vi "bumper b.vi"() -> ()   [LabVIEW 2013]
uses:
  <vilib>/NXT/Subs/MotorOutput.ctl
  <vilib>/NXT/Block Support/NXT_InputPort.ctl
panel:
  out "Output Ports (A & B) 34":T1=4 items=["Port A"=0, "Port B"=1, "Port C"=2, "Ports A & B"=4, "Ports A & C"=5, "Ports B & C"=6, "All Ports"=3]
  out "Output Port (All Ports) 15":T1=3 items=["Port A"=0, "Port B"=1, "Port C"=2, "Ports A & B"=4, "Ports A & C"=5, "Ports B & C"=6, "All Ports"=3]
  out "Output Ports (A & B) 33":T1=4 items=["Port A"=0, "Port B"=1, "Port C"=2, "Ports A & B"=4, "Ports A & C"=5, "Ports B & C"=6, "All Ports"=3]
  out "Output Ports (A & B) 32":T1=4 items=["Port A"=0, "Port B"=1, "Port C"=2, "Ports A & B"=4, "Ports A & C"=5, "Ports B & C"=6, "All Ports"=3]
  out "Output Port (All Ports) 14":T1=3 items=["Port A"=0, "Port B"=1, "Port C"=2, "Ports A & B"=4, "Ports A & C"=5, "Ports B & C"=6, "All Ports"=3]
  out "Output Ports (A & B) 31":T1=4 items=["Port A"=0, "Port B"=1, "Port C"=2, "Ports A & B"=4, "Ports A & C"=5, "Ports B & C"=6, "All Ports"=3]
  out "Output Ports (A & B) 30":T1=4 items=["Port A"=0, "Port B"=1, "Port C"=2, "Ports A & B"=4, "Ports A & C"=5, "Ports B & C"=6, "All Ports"=3]
  out "Output Port (All Ports) 13":T1=3 items=["Port A"=0, "Port B"=1, "Port C"=2, "Ports A & B"=4, "Ports A & C"=5, "Ports B & C"=6, "All Ports"=3]
  out "Output Ports (A & B) 29":T1=4 items=["Port A"=0, "Port B"=1, "Port C"=2, "Ports A & B"=4, "Ports A & C"=5, "Ports B & C"=6, "All Ports"=3]
  out "Output Ports (A & B) 28":T1=4 items=["Port A"=0, "Port B"=1, "Port C"=2, "Ports A & B"=4, "Ports A & C"=5, "Ports B & C"=6, "All Ports"=3]
  out "Output Port (All Ports) 12":T1=3 items=["Port A"=0, "Port B"=1, "Port C"=2, "Ports A & B"=4, "Ports A & C"=5, "Ports B & C"=6, "All Ports"=3]
  out "Output Ports (A & B) 27":T1=4 items=["Port A"=0, "Port B"=1, "Port C"=2, "Ports A & B"=4, "Ports A & C"=5, "Ports B & C"=6, "All Ports"=3]
  out "Output Ports (A & B) 26":T1=4 items=["Port A"=0, "Port B"=1, "Port C"=2, "Ports A & B"=4, "Ports A & C"=5, "Ports B & C"=6, "All Ports"=3]
  out "Output Port (All Ports) 11":T1=3 items=["Port A"=0, "Port B"=1, "Port C"=2, "Ports A & B"=4, "Ports A & C"=5, "Ports B & C"=6, "All Ports"=3]
  out "Output Ports (A & B) 25":T1=4 items=["Port A"=0, "Port B"=1, "Port C"=2, "Ports A & B"=4, "Ports A & C"=5, "Ports B & C"=6, "All Ports"=3]
  out "Output Ports (A & B) 24":T1=4 items=["Port A"=0, "Port B"=1, "Port C"=2, "Ports A & B"=4, "Ports A & C"=5, "Ports B & C"=6, "All Ports"=3]
  out "Output Port (All Ports) 10":T1=3 items=["Port A"=0, "Port B"=1, "Port C"=2, "Ports A & B"=4, "Ports A & C"=5, "Ports B & C"=6, "All Ports"=3]
  out "Output Ports (A & B) 23":T1=4 items=["Port A"=0, "Port B"=1, "Port C"=2, "Ports A & B"=4, "Ports A & C"=5, "Ports B & C"=6, "All Ports"=3]
  out "Output Ports (A & B) 22":T1=4 items=["Port A"=0, "Port B"=1, "Port C"=2, "Ports A & B"=4, "Ports A & C"=5, "Ports B & C"=6, "All Ports"=3]
  out "Output Port (All Ports) 9":T1=3 items=["Port A"=0, "Port B"=1, "Port C"=2, "Ports A & B"=4, "Ports A & C"=5, "Ports B & C"=6, "All Ports"=3]
  out "Output Ports (A & B) 21":T1=4 items=["Port A"=0, "Port B"=1, "Port C"=2, "Ports A & B"=4, "Ports A & C"=5, "Ports B & C"=6, "All Ports"=3]
  out "Output Ports (A & B) 20":T1=4 items=["Port A"=0, "Port B"=1, "Port C"=2, "Ports A & B"=4, "Ports A & C"=5, "Ports B & C"=6, "All Ports"=3]
  out "Output Port (All Ports) 8":T1=3 items=["Port A"=0, "Port B"=1, "Port C"=2, "Ports A & B"=4, "Ports A & C"=5, "Ports B & C"=6, "All Ports"=3]
  out "Output Ports (A & B) 19":T1=4 items=["Port A"=0, "Port B"=1, "Port C"=2, "Ports A & B"=4, "Ports A & C"=5, "Ports B & C"=6, "All Ports"=3]
  out "Output Ports (A & B) 18":T1=4 items=["Port A"=0, "Port B"=1, "Port C"=2, "Ports A & B"=4, "Ports A & C"=5, "Ports B & C"=6, "All Ports"=3]
  out "Output Port (All Ports) 7":T1=3 items=["Port A"=0, "Port B"=1, "Port C"=2, "Ports A & B"=4, "Ports A & C"=5, "Ports B & C"=6, "All Ports"=3]
  out "Output Ports (A & B) 17":T1=4 items=["Port A"=0, "Port B"=1, "Port C"=2, "Ports A & B"=4, "Ports A & C"=5, "Ports B & C"=6, "All Ports"=3]
  out "Output Ports (A & B) 16":T1=4 items=["Port A"=0, "Port B"=1, "Port C"=2, "Ports A & B"=4, "Ports A & C"=5, "Ports B & C"=6, "All Ports"=3]
  out "Output Port (All Ports) 6":T1=3 items=["Port A"=0, "Port B"=1, "Port C"=2, "Ports A & B"=4, "Ports A & C"=5, "Ports B & C"=6, "All Ports"=3]
  out "Output Ports (A & B) 15":T1=4 items=["Port A"=0, "Port B"=1, "Port C"=2, "Ports A & B"=4, "Ports A & C"=5, "Ports B & C"=6, "All Ports"=3]
  out "Output Ports (A & B) 14":T1=4 items=["Port A"=0, "Port B"=1, "Port C"=2, "Ports A & B"=4, "Ports A & C"=5, "Ports B & C"=6, "All Ports"=3]
  out "Output Port (All Ports) 5":T1=3 items=["Port A"=0, "Port B"=1, "Port C"=2, "Ports A & B"=4, "Ports A & C"=5, "Ports B & C"=6, "All Ports"=3]
  out "Output Ports (A & B) 13":T1=4 items=["Port A"=0, "Port B"=1, "Port C"=2, "Ports A & B"=4, "Ports A & C"=5, "Ports B & C"=6, "All Ports"=3]
  out "Output Ports (A & B) 9":T1=4 items=["Port A"=0, "Port B"=1, "Port C"=2, "Ports A & B"=4, "Ports A & C"=5, "Ports B & C"=6, "All Ports"=3]
  out "Output Port (All Ports) 4":T1=3 items=["Port A"=0, "Port B"=1, "Port C"=2, "Ports A & B"=4, "Ports A & C"=5, "Ports B & C"=6, "All Ports"=3]
  out "Output Ports (A & B) 11":T1=4 items=["Port A"=0, "Port B"=1, "Port C"=2, "Ports A & B"=4, "Ports A & C"=5, "Ports B & C"=6, "All Ports"=3]
  out "Output Port (All Ports) 3":T1=3 items=["Port A"=0, "Port B"=1, "Port C"=2, "Ports A & B"=4, "Ports A & C"=5, "Ports B & C"=6, "All Ports"=3]
  out "Output Ports (A & B) 12":T1=4 items=["Port A"=0, "Port B"=1, "Port C"=2, "Ports A & B"=4, "Ports A & C"=5, "Ports B & C"=6, "All Ports"=3]
  out "Output Ports (A & B) 10":T1=4 items=["Port A"=0, "Port B"=1, "Port C"=2, "Ports A & B"=4, "Ports A & C"=5, "Ports B & C"=6, "All Ports"=3]
  out "Output Ports (A & B) 5":T1=4 items=["Port A"=0, "Port B"=1, "Port C"=2, "Ports A & B"=4, "Ports A & C"=5, "Ports B & C"=6, "All Ports"=3]
  out "touch right":bool
  out "touch left":bool
  in  "threshold steer":dbl=0.2
  out "norm dist":dbl
  out "right dist":i16
  out "left dist":i16
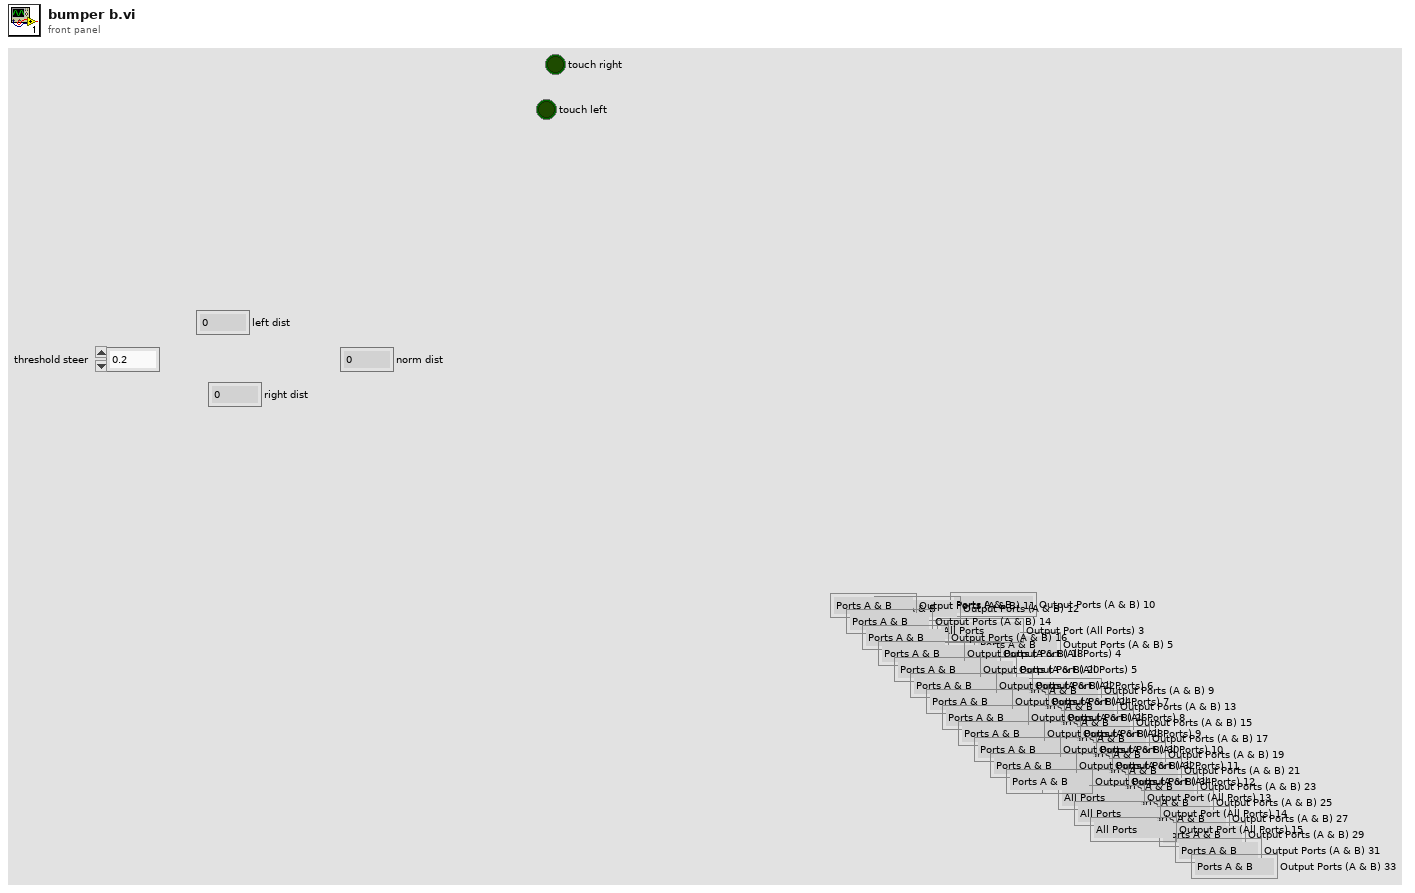
[diagram p1: front panel]
types:
  T1 = typedef "MotorOutput.ctl" = u8
  T2 = typedef "NXT_InputPort.ctl" = u32
  T3 = typedef "LVHSConnector.ctl" = refnum<class "BrickReference.lvclass">
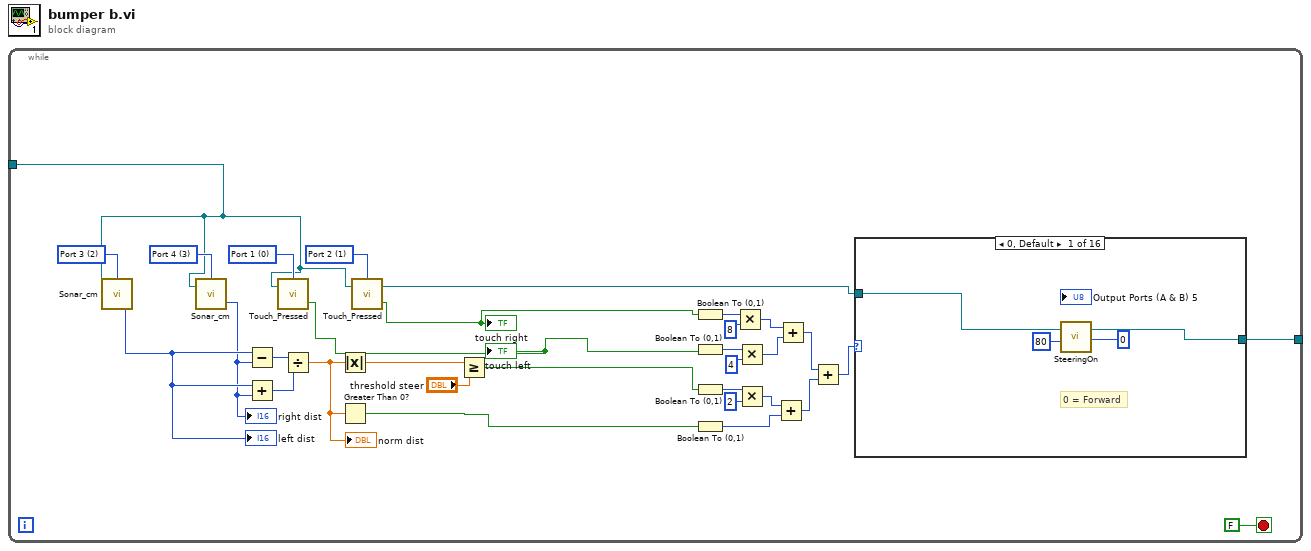
[diagram p0: block diagram]
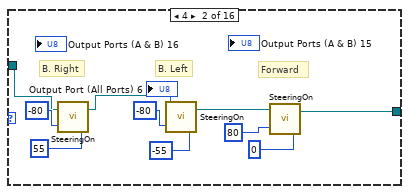
[diagram p2: hidden frame]
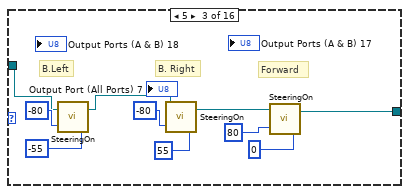
[diagram p3: hidden frame]
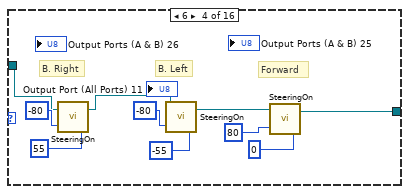
[diagram p4: hidden frame]
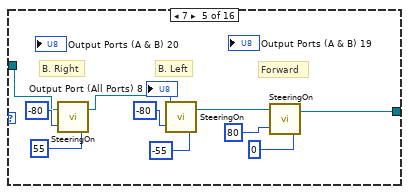
[diagram p5: hidden frame]
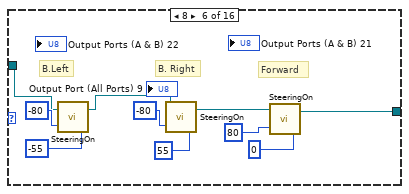
[diagram p6: hidden frame]
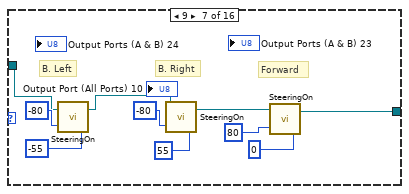
[diagram p7: hidden frame]
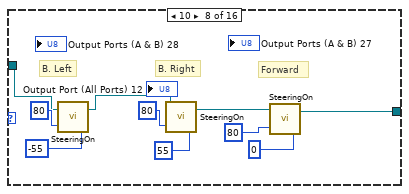
[diagram p8: hidden frame]
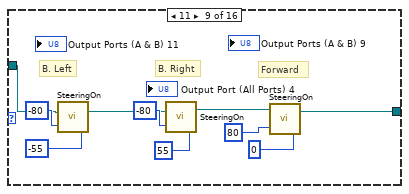
[diagram p9: hidden frame]
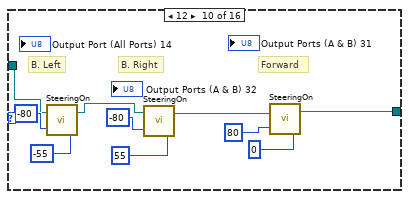
[diagram p10: hidden frame]
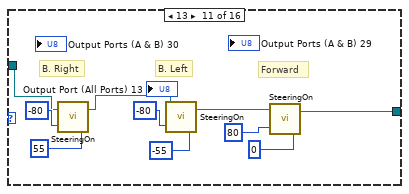
[diagram p11: hidden frame]
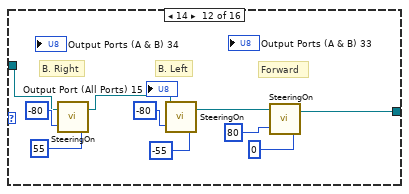
[diagram p12: hidden frame]
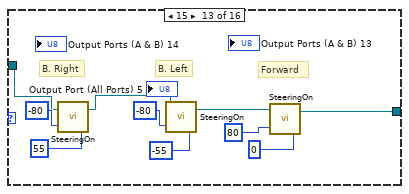
[diagram p13: hidden frame]
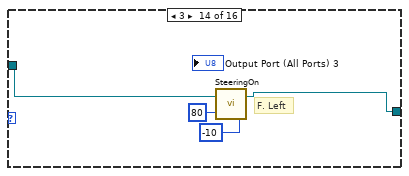
[diagram p14: hidden frame]
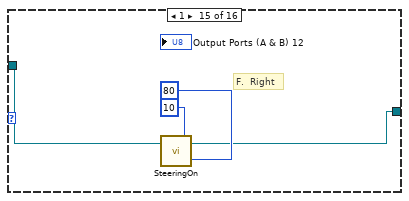
[diagram p15: hidden frame]
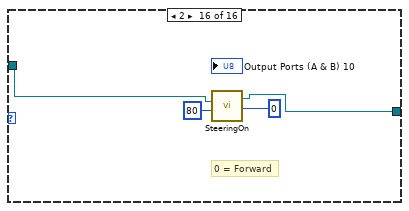
[diagram p16: hidden frame]
diagram:
  n1 = while {
    tunnel: [w7] -> _
    tunnel: [w1] -> _
    stop <- FALSE stop-if-true
    w22 = T2 1 items=["Port 1", "Port 2", "Port 3", "Port 4"] ("Port (Port 1)")
    w23 = T2 0 items=["Port 1", "Port 2", "Port 3", "Port 4"] ("Port (Port 1)")
    w31 = T2 3 items=["Port 1", "Port 2", "Port 3", "Port 4"] ("Port (Port 4)")
    w32 = T2 2 items=["Port 1", "Port 2", "Port 3", "Port 4"] ("Port (Port 4)")
    n2 = call <vilib>:"Sonar_cm.vi"("Port (Port 4)"=w32) -> ("Distance (cm)"=w30:i16, "NXT/EV3"=w1:T3)  [unwired: 2 in]
    "left dist" <- w30
    n3 = call <vilib>:"Sonar_cm.vi"("NXT/EV3"=w1, "Port (Port 4)"=w31) -> ("Distance (cm)"=w29:i16)  [unwired: 1 in, 1 out]
    "right dist" <- w29
    n4 = Subtract(x=w30, y=w29) -> (x-y=w28:i16)
    n5 = Add(x=w30, y=w29) -> (x+y=w27:i16)
    n6 = call <vilib>:"Touch_Pressed.vi"("NXT/EV3"=w1, "Port (Port 1)"=w23) -> ("Yes / No"=w4:bool)  [unwired: 1 in, 1 out]
    "touch left" <- w4
    n7 = Divide(x=w28, y=w27) -> (x/y=w24:dbl)
    "norm dist" <- w24
    n8 = Absolute Value(x=w24) -> (abs(x)=w26:dbl)
    n9 = Greater Than 0?(x=w24) -> (x > 0?=w9:bool)
    n10 = call <vilib>:"Touch_Pressed.vi"("NXT/EV3"=w1, "Port (Port 1)"=w22) -> ("Yes / No"=w3:bool, "NXT/EV3"=w2:T3)  [unwired: 1 in]
    "touch right" <- w3
    n11 = Greater Or Equal?(x=w26, y="threshold steer") -> (x >= y?=w8:bool)
    n12 = Boolean To (0,1)(Boolean=w3) -> (0, 1=w17:i16)
    n13 = Boolean To (0,1)(Boolean=w4) -> (0, 1=w16:i16)
    n14 = Boolean To (0,1)(Boolean=w8) -> (0, 1=w21:i16)
    n15 = Boolean To (0,1)(Boolean=w9) -> (0, 1=w11:i16)
    n16 = Multiply(x=w17, y=i16 8) -> (x*y=w14:i16)
    n17 = Multiply(x=w16, y=i16 4) -> (x*y=w13:i16)
    n18 = Multiply(x=w21, y=i16 2) -> (x*y=w12:i16)
    n19 = Add(x=w12, y=w11) -> (x+y=w10:i16)
    n20 = Add(x=w14, y=w13) -> (x+y=w15:i16)
    n21 = Add(x=w15, y=w10) -> (x+y=w5:i16)
    n22 = case shown="0, Default" w5 {
      tunnel: w2 -> [w34 w40 w50 w60 w70 w80 w90 w100 w110 w120 w130 w140 w150 w158 w162 w166]
      tunnel: [w33 w37 w47 w57 w67 w77 w87 w97 w107 w117 w127 w137 w147 w157 w161 w165] -> w7
      frame 0, Default {
        # "0 = Forward"
        n23 = call <vilib>:"SteeringOn.vi"("Power (75)"=80, "Steering (100)"=0, "NXT/EV3"=w34) -> ("NXT/EV3"=w33:T3)  [unwired: 1 in]
      }
      frame 4 {
        # "Forward"
        # "B. Left"
        # "B. Right"
        n24 = call <vilib>:"SteeringOn.vi"("Power (75)"=-80, "Steering (100)"=55, "NXT/EV3"=w40) -> ("NXT/EV3"=w39:T3)  [unwired: 1 in]
        n25 = call <vilib>:"SteeringOn.vi"("Power (75)"=-80, "Steering (100)"=-55, "NXT/EV3"=w39) -> ("NXT/EV3"=w38:T3)  [unwired: 1 in]
        n26 = call <vilib>:"SteeringOn.vi"("Power (75)"=80, "Steering (100)"=0, "NXT/EV3"=w38) -> ("NXT/EV3"=w37:T3)  [unwired: 1 in]
      }
      frame 5 {
        # "Forward"
        # "B. Right"
        # "B.Left"
        n27 = call <vilib>:"SteeringOn.vi"("Power (75)"=-80, "Steering (100)"=-55, "NXT/EV3"=w50) -> ("NXT/EV3"=w49:T3)  [unwired: 1 in]
        n28 = call <vilib>:"SteeringOn.vi"("Power (75)"=-80, "Steering (100)"=55, "NXT/EV3"=w49) -> ("NXT/EV3"=w48:T3)  [unwired: 1 in]
        n29 = call <vilib>:"SteeringOn.vi"("Power (75)"=80, "Steering (100)"=0, "NXT/EV3"=w48) -> ("NXT/EV3"=w47:T3)  [unwired: 1 in]
      }
      frame 6 {
        # "Forward"
        # "B. Left"
        # "B. Right"
        n30 = call <vilib>:"SteeringOn.vi"("Power (75)"=-80, "Steering (100)"=55, "NXT/EV3"=w60) -> ("NXT/EV3"=w59:T3)  [unwired: 1 in]
        n31 = call <vilib>:"SteeringOn.vi"("Power (75)"=-80, "Steering (100)"=-55, "NXT/EV3"=w59) -> ("NXT/EV3"=w58:T3)  [unwired: 1 in]
        n32 = call <vilib>:"SteeringOn.vi"("Power (75)"=80, "Steering (100)"=0, "NXT/EV3"=w58) -> ("NXT/EV3"=w57:T3)  [unwired: 1 in]
      }
      frame 7 {
        # "Forward"
        # "B. Left"
        # "B. Right"
        n33 = call <vilib>:"SteeringOn.vi"("Power (75)"=-80, "Steering (100)"=55, "NXT/EV3"=w70) -> ("NXT/EV3"=w69:T3)  [unwired: 1 in]
        n34 = call <vilib>:"SteeringOn.vi"("Power (75)"=-80, "Steering (100)"=-55, "NXT/EV3"=w69) -> ("NXT/EV3"=w68:T3)  [unwired: 1 in]
        n35 = call <vilib>:"SteeringOn.vi"("Power (75)"=80, "Steering (100)"=0, "NXT/EV3"=w68) -> ("NXT/EV3"=w67:T3)  [unwired: 1 in]
      }
      frame 8 {
        # "Forward"
        # "B. Right"
        # "B.Left"
        n36 = call <vilib>:"SteeringOn.vi"("Power (75)"=-80, "Steering (100)"=-55, "NXT/EV3"=w80) -> ("NXT/EV3"=w79:T3)  [unwired: 1 in]
        n37 = call <vilib>:"SteeringOn.vi"("Power (75)"=-80, "Steering (100)"=55, "NXT/EV3"=w79) -> ("NXT/EV3"=w78:T3)  [unwired: 1 in]
        n38 = call <vilib>:"SteeringOn.vi"("Power (75)"=80, "Steering (100)"=0, "NXT/EV3"=w78) -> ("NXT/EV3"=w77:T3)  [unwired: 1 in]
      }
      frame 9 {
        # "Forward"
        # "B. Right"
        # "B. Left"
        n39 = call <vilib>:"SteeringOn.vi"("Power (75)"=-80, "Steering (100)"=-55, "NXT/EV3"=w90) -> ("NXT/EV3"=w89:T3)  [unwired: 1 in]
        n40 = call <vilib>:"SteeringOn.vi"("Power (75)"=-80, "Steering (100)"=55, "NXT/EV3"=w89) -> ("NXT/EV3"=w88:T3)  [unwired: 1 in]
        n41 = call <vilib>:"SteeringOn.vi"("Power (75)"=80, "Steering (100)"=0, "NXT/EV3"=w88) -> ("NXT/EV3"=w87:T3)  [unwired: 1 in]
      }
      frame 10 {
        # "Forward"
        # "B. Right"
        # "B. Left"
        n42 = call <vilib>:"SteeringOn.vi"("Power (75)"=80, "Steering (100)"=-55, "NXT/EV3"=w100) -> ("NXT/EV3"=w99:T3)  [unwired: 1 in]
        n43 = call <vilib>:"SteeringOn.vi"("Power (75)"=80, "Steering (100)"=55, "NXT/EV3"=w99) -> ("NXT/EV3"=w98:T3)  [unwired: 1 in]
        n44 = call <vilib>:"SteeringOn.vi"("Power (75)"=80, "Steering (100)"=0, "NXT/EV3"=w98) -> ("NXT/EV3"=w97:T3)  [unwired: 1 in]
      }
      frame 11 {
        # "Forward"
        # "B. Right"
        # "B. Left"
        n45 = call <vilib>:"SteeringOn.vi"("Power (75)"=-80, "Steering (100)"=-55, "NXT/EV3"=w110) -> ("NXT/EV3"=w109:T3)  [unwired: 1 in]
        n46 = call <vilib>:"SteeringOn.vi"("Power (75)"=-80, "Steering (100)"=55, "NXT/EV3"=w109) -> ("NXT/EV3"=w108:T3)  [unwired: 1 in]
        n47 = call <vilib>:"SteeringOn.vi"("Power (75)"=80, "Steering (100)"=0, "NXT/EV3"=w108) -> ("NXT/EV3"=w107:T3)  [unwired: 1 in]
      }
      frame 12 {
        # "B. Right"
        # "Forward"
        # "B. Left"
        n48 = call <vilib>:"SteeringOn.vi"("Power (75)"=-80, "Steering (100)"=-55, "NXT/EV3"=w120) -> ("NXT/EV3"=w119:T3)  [unwired: 1 in]
        n49 = call <vilib>:"SteeringOn.vi"("Power (75)"=-80, "Steering (100)"=55, "NXT/EV3"=w119) -> ("NXT/EV3"=w118:T3)  [unwired: 1 in]
        n50 = call <vilib>:"SteeringOn.vi"("Power (75)"=80, "Steering (100)"=0, "NXT/EV3"=w118) -> ("NXT/EV3"=w117:T3)  [unwired: 1 in]
      }
      frame 13 {
        # "Forward"
        # "B. Left"
        # "B. Right"
        n51 = call <vilib>:"SteeringOn.vi"("Power (75)"=-80, "Steering (100)"=55, "NXT/EV3"=w130) -> ("NXT/EV3"=w129:T3)  [unwired: 1 in]
        n52 = call <vilib>:"SteeringOn.vi"("Power (75)"=-80, "Steering (100)"=-55, "NXT/EV3"=w129) -> ("NXT/EV3"=w128:T3)  [unwired: 1 in]
        n53 = call <vilib>:"SteeringOn.vi"("Power (75)"=80, "Steering (100)"=0, "NXT/EV3"=w128) -> ("NXT/EV3"=w127:T3)  [unwired: 1 in]
      }
      frame 14 {
        # "Forward"
        # "B. Left"
        # "B. Right"
        n54 = call <vilib>:"SteeringOn.vi"("Power (75)"=-80, "Steering (100)"=55, "NXT/EV3"=w140) -> ("NXT/EV3"=w139:T3)  [unwired: 1 in]
        n55 = call <vilib>:"SteeringOn.vi"("Power (75)"=-80, "Steering (100)"=-55, "NXT/EV3"=w139) -> ("NXT/EV3"=w138:T3)  [unwired: 1 in]
        n56 = call <vilib>:"SteeringOn.vi"("Power (75)"=80, "Steering (100)"=0, "NXT/EV3"=w138) -> ("NXT/EV3"=w137:T3)  [unwired: 1 in]
      }
      frame 15 {
        # "Forward"
        # "B. Left"
        # "B. Right"
        n57 = call <vilib>:"SteeringOn.vi"("Power (75)"=-80, "Steering (100)"=55, "NXT/EV3"=w150) -> ("NXT/EV3"=w149:T3)  [unwired: 1 in]
        n58 = call <vilib>:"SteeringOn.vi"("Power (75)"=-80, "Steering (100)"=-55, "NXT/EV3"=w149) -> ("NXT/EV3"=w148:T3)  [unwired: 1 in]
        n59 = call <vilib>:"SteeringOn.vi"("Power (75)"=80, "Steering (100)"=0, "NXT/EV3"=w148) -> ("NXT/EV3"=w147:T3)  [unwired: 1 in]
      }
      frame 3 {
        # "F. Left"
        n60 = call <vilib>:"SteeringOn.vi"("Power (75)"=80, "Steering (100)"=-10, "NXT/EV3"=w158) -> ("NXT/EV3"=w157:T3)  [unwired: 1 in]
      }
      frame 1 {
        # "F.  Right"
        n61 = call <vilib>:"SteeringOn.vi"("Power (75)"=80, "Steering (100)"=10, "NXT/EV3"=w162) -> ("NXT/EV3"=w161:T3)  [unwired: 1 in]
      }
      frame 2 {
        # "0 = Forward"
        n62 = call <vilib>:"SteeringOn.vi"("Power (75)"=80, "Steering (100)"=0, "NXT/EV3"=w166) -> ("NXT/EV3"=w165:T3)  [unwired: 1 in]
      }
    }
  }
